vi "写入参数.vi"(7 "写入参数":T1(ring), 8 "error in (no error)":errorcluster, 11 "写入值":sgl) -> (0 "error out":errorcluster)   [LabVIEW 2016, in "一代CodMn.lvlib"]
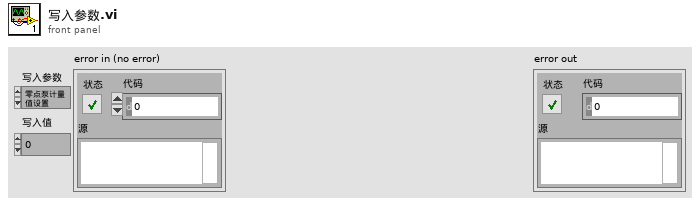
[diagram p1: front panel]
types:
  T1 = enum16{"零点泵计量值设置", "零点滴定值设置", "标度泵计量值设置", "标度滴定值设定", "标液浓度设置"}
  T2 = enum16{"open", "close", "readHR", "writeHR", "readCoil", "writeCoil"}
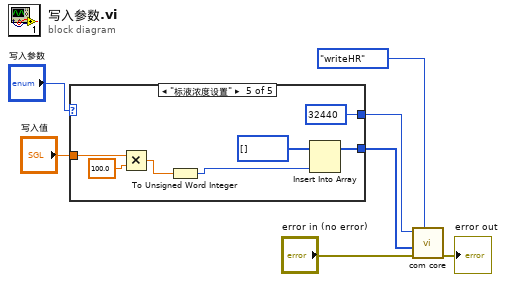
[diagram p0: block diagram]
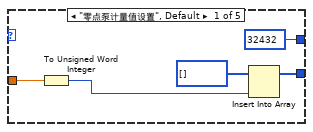
[diagram p2: hidden frame]
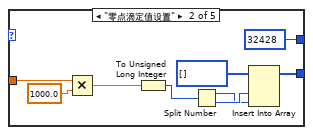
[diagram p3: hidden frame]
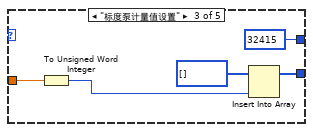
[diagram p4: hidden frame]
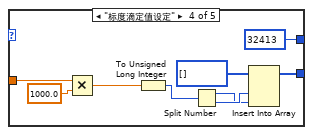
[diagram p5: hidden frame]
diagram:
  n1 = case shown="\"标液浓度设置\"" "写入参数" {
    tunnel: [u16 32432 ("starting address") u16 32428 ("starting address") u16 32415 ("starting address") u16 32413 ("starting address") u16 32440 ("starting address")] -> w5
    tunnel: "写入值" -> [w11 w20 w24 w28 w38]
    tunnel: [w8 w15 w23 w27 w39] -> w3
    frame "零点泵计量值设置", Default {
      n2 = To Unsigned Word Integer(number=w11) -> (unsigned 16bit integer=w9:u16)
      n3 = Insert Into Array(array=u16[] [] ("HR values"), new element=w9) -> (w8:u16[])  [unwired: 1 in]
    }
    frame "零点滴定值设置" {
      n4 = Multiply(x=w20, y=sgl 1000.0) -> (x*y=w18:sgl)
      n5 = To Unsigned Long Integer(number=w18) -> (unsigned 32bit integer=w17:u32)
      n6 = Split Number(x=w17) -> (hi(x)=w13:u16, lo(x)=w14:u16)
      n7 = Insert Into Array(array=u16[] [] ("HR values"), new element #1=w14, new element #2=w13) -> (w15:u16[])  [unwired: 1 in]
    }
    frame "标度泵计量值设置" {
      n8 = To Unsigned Word Integer(number=w24) -> (unsigned 16bit integer=w25:u16)
      n9 = Insert Into Array(array=u16[] [] ("HR values"), new element=w25) -> (w23:u16[])  [unwired: 1 in]
    }
    frame "标度滴定值设定" {
      n10 = Multiply(x=w28, y=sgl 1000.0) -> (x*y=w33:sgl)
      n11 = To Unsigned Long Integer(number=w33) -> (unsigned 32bit integer=w32:u32)
      n12 = Split Number(x=w32) -> (hi(x)=w29:u16, lo(x)=w30:u16)
      n13 = Insert Into Array(array=u16[] [] ("HR values"), new element #1=w30, new element #2=w29) -> (w27:u16[])  [unwired: 1 in]
    }
    frame "标液浓度设置" {
      n14 = Multiply(x=w38, y=sgl 100.0) -> (x*y=w37:sgl)
      n15 = To Unsigned Word Integer(number=w37) -> (unsigned 16bit integer=w36:u16)
      n16 = Insert Into Array(array=u16[] [] ("HR values"), new element=w36) -> (w39:u16[])  [unwired: 1 in]
    }
  }
  n17 = call "com core.vi"("功能"=T2."writeHR", "error in (no error)"="error in (no error)", "HR values"=w3, "starting address"=w5) -> ("error out"=→"error out":errorcluster)  [unwired: 5 in, 2 out]
